vi "cluster_from_ini_file.vi"(8 "error in (no error)":errorcluster, 10 "dataType":variant, 11 "iniFilePath":path) -> (0 "error out":errorcluster, 2 "dataValue":variant)   [LabVIEW 2015, in "ini_work_Library.lvlib"]
doc: "Created by Artem Shevelev\nshevelev.pro\nartem@shevelev.pro\nLabVIEW Portal: https://labviewportal.org/memberlist.php?mode=viewprofile&u=2340"
uses:
  ini_work_Library.lvlib
  <vilib>/Utility/config.llb/NI_LVConfig.lvlib
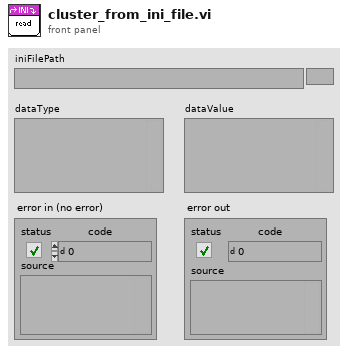
[diagram p1: front panel]
types:
  T1 = typedef "NI_LVConfig.lvlib/Config Data RefNum.ctl" = refnum<k1>
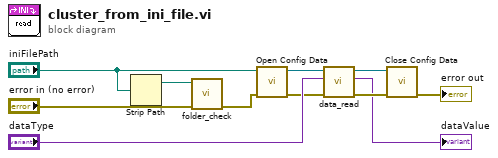
[diagram p0: block diagram]
diagram:
  n1 = Strip Path(path="iniFilePath") -> (stripped path=w3:path)  [unwired: 1 out]
  n2 = call "folder_check.vi"("error in (no error)"="error in (no error)", "stripped path"=w3) -> ("error out"=w1:errorcluster)  [unwired: 9 in]
  n3 = call <vilib>:"Open Config Data.vi"("error in (no error)"=w1, "configuration file path"="iniFilePath") -> ("error out"=w8:errorcluster, "refnum"=w10:T1)  [unwired: 7 in, 1 out]
  n4 = call "data_read.vi"("error in (no error)"=w8, "dataContainer"="dataType", "ini_file_refnum"=w10) -> ("error out"=w6:errorcluster, "dataValue"=→"dataValue":variant, "ini_file_refnum_out"=w7:T1)  [unwired: 6 in]
  n5 = call <vilib>:"Close Config Data.vi"("error in (no error)"=w6, "refnum"=w7) -> ("error out"=→"error out":errorcluster)  [unwired: 8 in, 1 out]
